vi "Fibonacci.vi"(7 "Memo":u32[](array[numeric]), 11 "n":u32) -> (3 "fib(n)":u32)   [LabVIEW 2013, in "Problem 2.lvlib"]
uses:
  Problem 2.lvlib
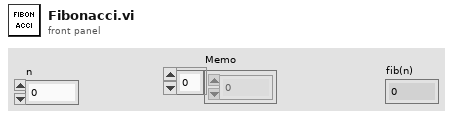
[diagram p1: front panel]
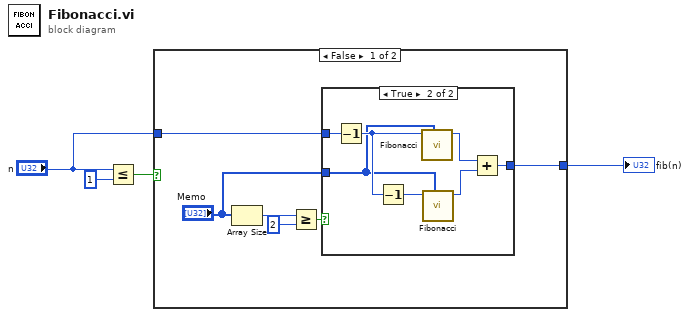
[diagram p0: block diagram]
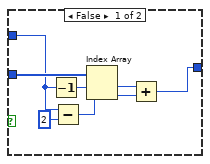
[diagram p2: hidden frame]
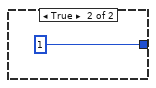
[diagram p3: hidden frame]
diagram:
  n1 = Less Or Equal?(x="n", y=u32 1) -> (x <= y?=w3:bool)
  n2 = case shown="False" w3 {
    tunnel: "n" -> [w10 _]
    tunnel: [w9 u32 1 ("y")] -> w1
    frame False {
      n3 = Array Size(array="Memo") -> (size(s)=w7:i32)
      n4 = Greater Or Equal?(x=w7, y=2) -> (x >= y?=w8:bool)
      n5 = case shown="True" w8 {
        tunnel: w10 -> [w15 w25]
        tunnel: [w11 w20] -> w9
        tunnel: "Memo" -> [w18 w19]
        frame False {
          n6 = Decrement(x=w15) -> (x-1=w17:u32)
          n7 = Subtract(x=w15, y=u32 2) -> (x-y=w16:u32)
          n8 = Index Array(array=w18, index #1=w17, index #2=w16) -> (element #1=w13:u32, element #2=w12:u32)
          n9 = Add(x=w13, y=w12) -> (x+y=w11:u32)
        }
        frame True {
          n10 = Decrement(x=w25) -> (x-1=w24:u32)
          n11 = Decrement(x=w24) -> (x-1=w23:u32)
          n12 = call "Fibonacci.vi"("Memo"=w19, "n"=w24) -> ("fib(n)"=w21:u32)  [unwired: 9 in]
          n13 = call "Fibonacci.vi"("Memo"=w19, "n"=w23) -> ("fib(n)"=w22:u32)  [unwired: 9 in]
          n14 = Add(x=w21, y=w22) -> (x+y=w20:u32)
        }
      }
    }
    frame True {
    }
  }
  "fib(n)" <- w1
